vi "ROS_Master_CloseAllServiceProviders.vi"(3 "Current Master":T1) -> ()   [LabVIEW 2012]
doc: "Closes all service providers"
uses:
  <userlib>/ROS for LabVIEW Software/ROS/Code/ROS_Master/ROS_Master.ctl
  <userlib>/ROS for LabVIEW Software/ROS/Code/ROS_Master/ROS_Topic.ctl
  <userlib>/ROS for LabVIEW Software/ROS/Code/ROS_Master/ROS_Node.ctl
  <userlib>/ROS for LabVIEW Software/ROS/Code/ROS_Master/ROS_Service.ctl
panel:
  out "Array":errorcluster[](array[cluster])
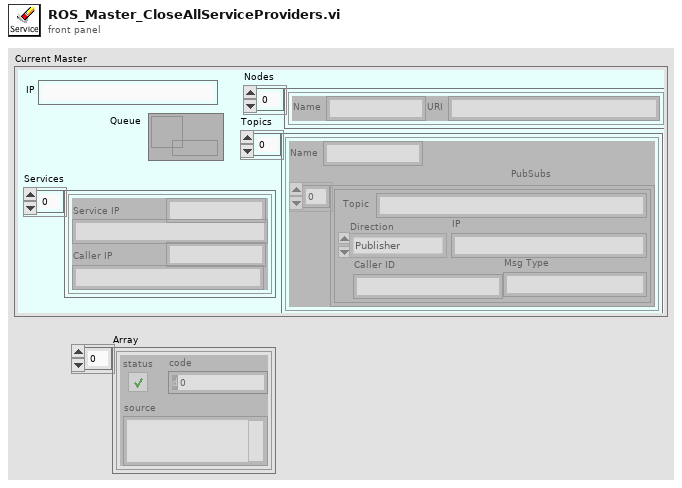
[diagram p1: front panel]
types:
  T1 = typedef "ROS_Master.ctl" = cluster{"IP":string, "Topics":cluster{"Name":string, "PubSubs":T2[]}[], "Nodes":T3[], "Services":T4[], "Queue":refnum<queue>}
  T2 = typedef "ROS_Topic.ctl" = cluster{"Caller ID":string, "IP":string, "Msg Type":string, "Direction":enum16{"Publisher", "Subscriber"}, "Topic":string}
  T3 = typedef "ROS_Node.ctl" = cluster{"Name":string, "URI":string}
  T4 = typedef "ROS_Service.ctl" = cluster{"Service":string, "Service IP":string, "Caller IP":string, "Caller ID":string}
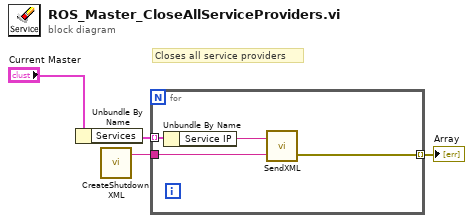
[diagram p0: block diagram]
diagram:
  # "Closes all service providers"
  n1 = Unbundle By Name("Current Master") -> ("Services"=w3:T4[])
  n2 = call <userlib>:"CreateShutdownXML.vi"() -> ("XML"=w2:string)  [unwired: 3 in]
  n3 = for {
    tunnel: w3 -> [w8] mode=indexing
    tunnel: w2 -> [w6]
    tunnel: [w5] -> w1 mode=indexing
    n4 = Unbundle By Name(w8) -> ("Service IP"=w7:string)
    n5 = call <userlib>:"SendXML.vi"("Send"=w6, "URI in"=w7) -> ("error out"=w5:errorcluster)  [unwired: 1 out]
  }
  "Array" <- w1
